vi "Write Analogue.vi"(8 "error in (no error)":errorcluster, 9 "output":bool, 10 "Channel index(0)":i32, 11 "Sim Fgen in":refnum<class "Sim Fgen.lvclass">) -> (0 "error out":errorcluster, 2 "Success?":bool, 3 "Sim Fgen out":refnum<class "Sim Fgen.lvclass">)   [LabVIEW 2025, in "Fgen.lvlib" / "Sim Fgen.lvclass"]
uses:
  Sim Fgen.lvclass
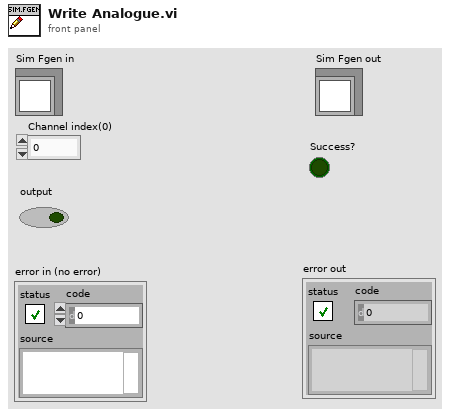
[diagram p1: front panel]
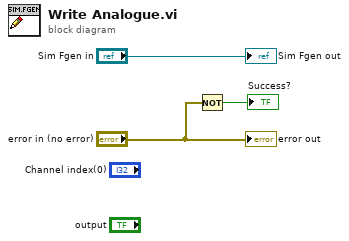
[diagram p0: block diagram]
diagram:
  n1 = Not(x="error in (no error)") -> (.not. x?=→"Success?":bool)
  "error out" <- "error in (no error)"
  "Sim Fgen out" <- "Sim Fgen in"
